vi "Example Play File 2.vi"() -> ()   [LabVIEW 2014]
uses:
  <vilib>/LabVIEW Universal Transcriptor/LabVIEW to Arduino Transcriptor/Transcriptors/System API/Serial println string.vi
  TMRpcm.lvlib
  <vilib>/LabVIEW Universal Transcriptor/LabVIEW Universal Transcriptor SD Card Library/LabVIEW Universal Transcriptor SD Card Library.lvlib
panel:
  out "Error Out":errorcluster
  in  "Error In":errorcluster
  # "max 8 characters together with file extension"
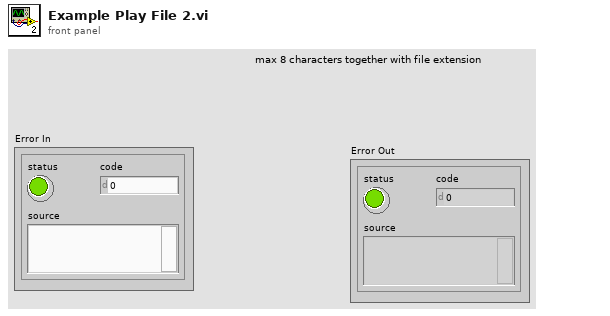
[diagram p1: front panel]
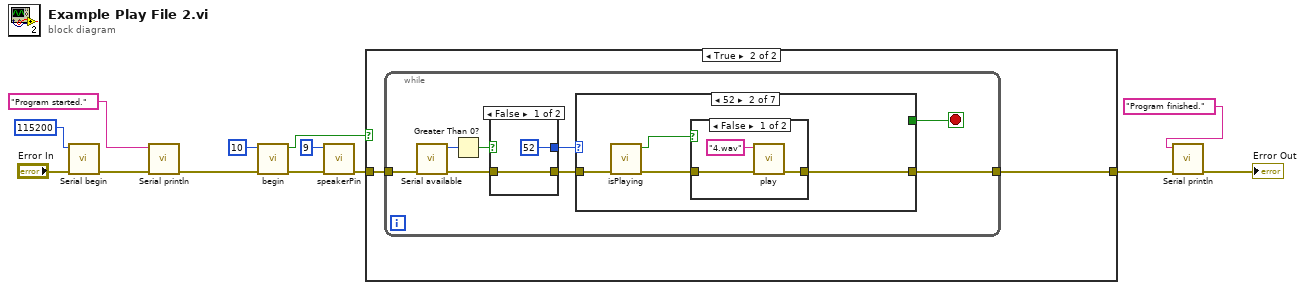
[diagram p0: block diagram]
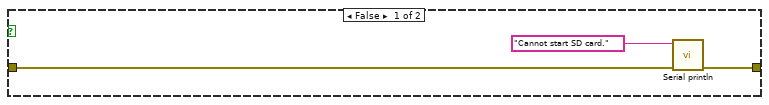
[diagram p2: hidden frame]
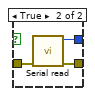
[diagram p3: hidden frame]
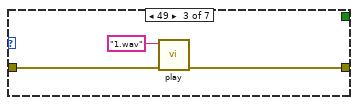
[diagram p6: hidden frame]
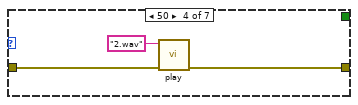
[diagram p7: hidden frame]
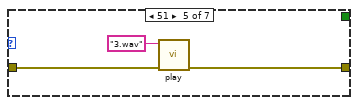
[diagram p8: hidden frame]
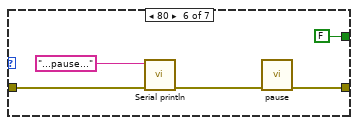
[diagram p9: hidden frame]
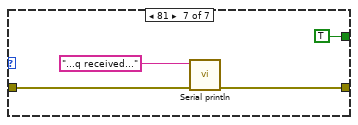
[diagram p10: hidden frame]
diagram:
  n1 = call <vilib>:"Serial begin.vi"("Error In"="Error In", "speed (Bd)"=115200) -> ("Error Out"=w12:errorcluster)  [unwired: 9 in]
  n2 = call-poly <vilib>:"Serial println.vi"("Error In"=w12, "string in"="Program started.") -> ("Error Out"=w8:errorcluster)  [unwired: 9 in]
  n3 = call <vilib>:"begin.vi"("Error In"=w8, "CS pin (optional)"=u8 10) -> ("Error Out"=w2:errorcluster, "success?"=w7:bool)  [unwired: 8 in]
  n4 = call "speakerPin.vi"("Error In"=w2, "speakerPin"=u8 9) -> ("Error Out"=w1:errorcluster)  [unwired: 9 in]
  n5 = case shown="True" w7 {
    tunnel: [w15 w18] -> w6
    tunnel: w1 -> [w16 w17]
    frame False {
      n6 = call-poly <vilib>:"Serial println.vi"("Error In"=w16, "string in"="Cannot start SD card.") -> ("Error Out"=w15:errorcluster)  [unwired: 9 in]
    }
    frame True {
      n7 = while {
        tunnel: w17 -> [w23]
        tunnel: [w19] -> w18
        stop <- w25 stop-if-true
        n8 = call <vilib>:"Serial available.vi"("Error In"=w23) -> ("Error Out"=w22:errorcluster, "available bytes"=w21:i32)  [unwired: 9 in]
        n9 = Greater Than 0?(x=w21) -> (x > 0?=w20:bool)
        n10 = case shown="False" w20 {
          tunnel: [w28 w31] -> w26
          tunnel: [52 ("data") w30] -> w24
          tunnel: w22 -> [w28 w29]
          frame False {
          }
          frame True {
            n11 = call <vilib>:"Serial read.vi"("Error In"=w29) -> ("Error Out"=w31:errorcluster, "data"=w30:i32)  [unwired: 9 in]
          }
        }
        n12 = case shown="52" w24 {
          tunnel: [w32 w34 w41 w44 w47 w54 w56] -> w19
          tunnel: w26 -> [w32 w36 w43 w45 w48 w52 w55]
          tunnel: [_ _ _ _ _ FALSE TRUE] -> w25
          frame Default {
          }
          frame 52 {
            n13 = call "isPlaying.vi"("Error In"=w36) -> ("Error Out"=w35:errorcluster, "isPlaying"=w33:bool)  [unwired: 9 in]
            n14 = case shown="False" w33 {
              tunnel: w35 -> [w39 w40]
              tunnel: [w37 w40] -> w34
              frame False {
                n15 = call "play.vi"("Error In"=w39, "filename"="4.wav") -> ("Error Out"=w37:errorcluster)  [unwired: 9 in]
              }
              frame True {
              }
            }
          }
          frame 49 {
            n16 = call "play.vi"("Error In"=w43, "filename"="1.wav") -> ("Error Out"=w41:errorcluster)  [unwired: 9 in]
          }
          frame 50 {
            n17 = call "play.vi"("Error In"=w45, "filename"="2.wav") -> ("Error Out"=w44:errorcluster)  [unwired: 9 in]
          }
          frame 51 {
            n18 = call "play.vi"("Error In"=w48, "filename"="3.wav") -> ("Error Out"=w47:errorcluster)  [unwired: 9 in]
          }
          frame 80 {
            n19 = call-poly <vilib>:"Serial println.vi"("Error In"=w52, "string in"="...pause...") -> ("Error Out"=w51:errorcluster)  [unwired: 9 in]
            n20 = call "pause.vi"("Error In"=w51) -> ("Error Out"=w54:errorcluster)  [unwired: 10 in]
          }
          frame 81 {
            n21 = call-poly <vilib>:"Serial println.vi"("Error In"=w55, "string in"="...q received...") -> ("Error Out"=w56:errorcluster)  [unwired: 9 in]
          }
        }
      }
    }
  }
  n22 = call-poly <vilib>:"Serial println.vi"("Error In"=w6, "string in"="Program finished.") -> ("Error Out"=→"Error Out":errorcluster)  [unwired: 9 in]
